vi "CRYUnflatten Data.vi"(11 "Unflatten data":string) -> (0 "Error?":bool, 2 "Datum":T2={"Name"="", "Curve"=[], "X data"=1, "Y data"=1, "Z data"=1, "X axis"=0, "Y axis"=1, "Z axis"=1, "X unit"="", "Y unit"="", "Z unit"="", "X dB ref"=1.0, "Y dB ref"=1.0, "Z dB ref"=1.0, "single val"=FALSE, "protected"=FALSE, "display X"=TRUE, "display Y"=FALSE, "display Z"=TRUE, "Test Info"="", "Step No."=0, "Plot Settings"={"Color"=0, "Interpolation"=0, "Point Style"=0, "Line Style"=0, "Point Color"=0, "Line Width"=0, "Bar Plot Style"=0, "Fill To"=0}, "AutoProtect"=FALSE} {"Z data" items=["dB", "Lin"]; "X data" items=["dB", "Lin"]; "Y data" items=["dB", "Lin"]; "Z dB ref" format="%.1f"; "Z axis" items=["Log", "Lin"]; "X dB ref" format="%.1f"; "X axis" items=["Log", "Lin"]; "Y axis" items=["Log", "Lin"]; "Y dB ref" format="%.1f"; "Curve"."z" format="%.2f"; "Curve"."y" format="%.2f"; "Curve"."x" format="%.2f"}, 3 "Header info":T1={"Data type"="Data            ", "Version"=1, "Dimensions"=0})   [LabVIEW 2013]
uses:
  Typedef Control/CRYData Cluster.ctl
  CRYCurveLibrary/Global/CRYCurve Library Global.vi
panel:
  # "-"
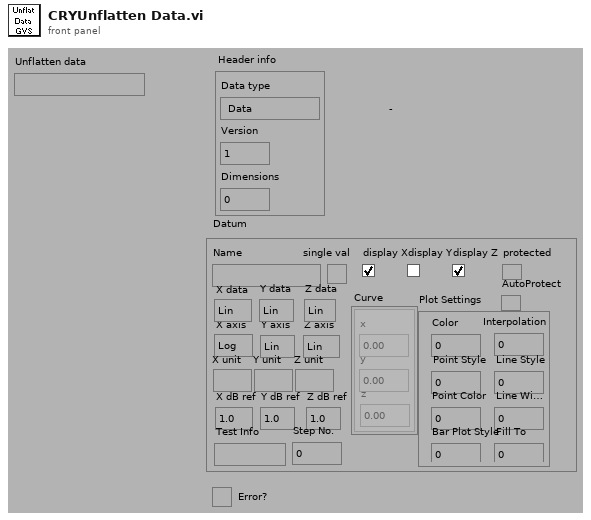
[diagram p1: front panel]
types:
  T1 = cluster{"Data type":string, "Version":u16, "Dimensions":u8}
  T2 = typedef "CRYData Cluster.ctl" = cluster{"Name":string, "Curve":cluster{"x":dbl, "y":dbl, "z":dbl}[], "X data":u16, "Y data":u16, "Z data":u16, "X axis":u16, "Y axis":u16, "Z axis":u16, "X unit":string, "Y unit":string, "Z unit":string, "X dB ref":dbl, "Y dB ref":dbl, "Z dB ref":dbl, "single val":bool, "protected":bool, "display X":bool, "display Y":bool, "display Z":bool, "Test Info":string, "Step No.":i32, "Plot Settings":cluster{"Color":u32, "Interpolation":u8, "Point Style":u8, "Line Style":u8, "Point Color":u32, "Line Width":u8, "Bar Plot Style":u8, "Fill To":i16}, "AutoProtect":bool}
  T3 = cluster{"Name":string, "Curve":cluster{"x":dbl, "y":dbl, "z":dbl}[], "X data":u16, "Y data":u16, "Z data":u16, "X axis":u16, "Y axis":u16, "Z axis":u16, "X unit":string, "Y unit":string, "Z unit":string, "X dB ref":dbl, "Y dB ref":dbl, "Z dB ref":dbl, "single val":bool, "protected":bool, "display X":bool, "display Y":bool, "display Z":bool, "Test Info":string, "Step No.":i32, "Plot Settings":cluster{"Color":u32, "Interpolation":u8, "Point Style":u8, "Line Style":u8, "Point Color":u32, "Line Width":u8, "Bar Plot Style":u8, "Fill To":i16}, "AutoProtect":bool}
  T4 = cluster{"unsigned byte array[0]":u8, "unsigned byte array[1]":u8, "unsigned byte array[2]":u8}
  T5 = cluster{"Name":string, "Curve":cluster{"x":dbl, "y":dbl, "z":dbl}[], "X data":u16, "Y data":u16, "Z data":u16, "X axis":u16, "Y axis":u16, "Z axis":u16, "X prefix":string, "Y prefix":string, "Z prefix":string, "X unit":string, "Y unit":string, "Z unit":string, "X dB ref":dbl, "Y dB ref":dbl, "Z dB ref":dbl}
  T6 = typedef "CRYData Cluster SC.ctl" = cluster{"Name":string, "Curve":cluster{"x":dbl, "y":dbl, "z":dbl}[], "X data":T7, "Y data":T7, "Z data":T7, "X axis":u16, "Y axis":u16, "Z axis":u16, "X unit":string, "Y unit":string, "Z unit":string, "X dB ref":dbl, "Y dB ref":dbl, "Z dB ref":dbl, "single val":bool, "protected":bool, "display X":bool, "display Y":bool, "display Z":bool, "Plot Settings":cluster{"Color":u32, "Interpolation":u8, "Point Style":u8, "Line Style":u8, "Point Color":u32, "Line Width":u8, "Bar Plot Style":u8, "Fill To":i16}, "Test Info":string}
  T7 = typedef "CRYAxis Unit Type.ctl" = u16
  T8 = cluster{"Color":u32, "Interpolation":u8, "Point Style":u8, "Line Style":u8, "Point Color":u32, "Line Width":u8, "Bar Plot Style":u8, "Fill To":i16}
  T9 = cluster{"substring":string, u16, "unsigned byte array[2]":u8}
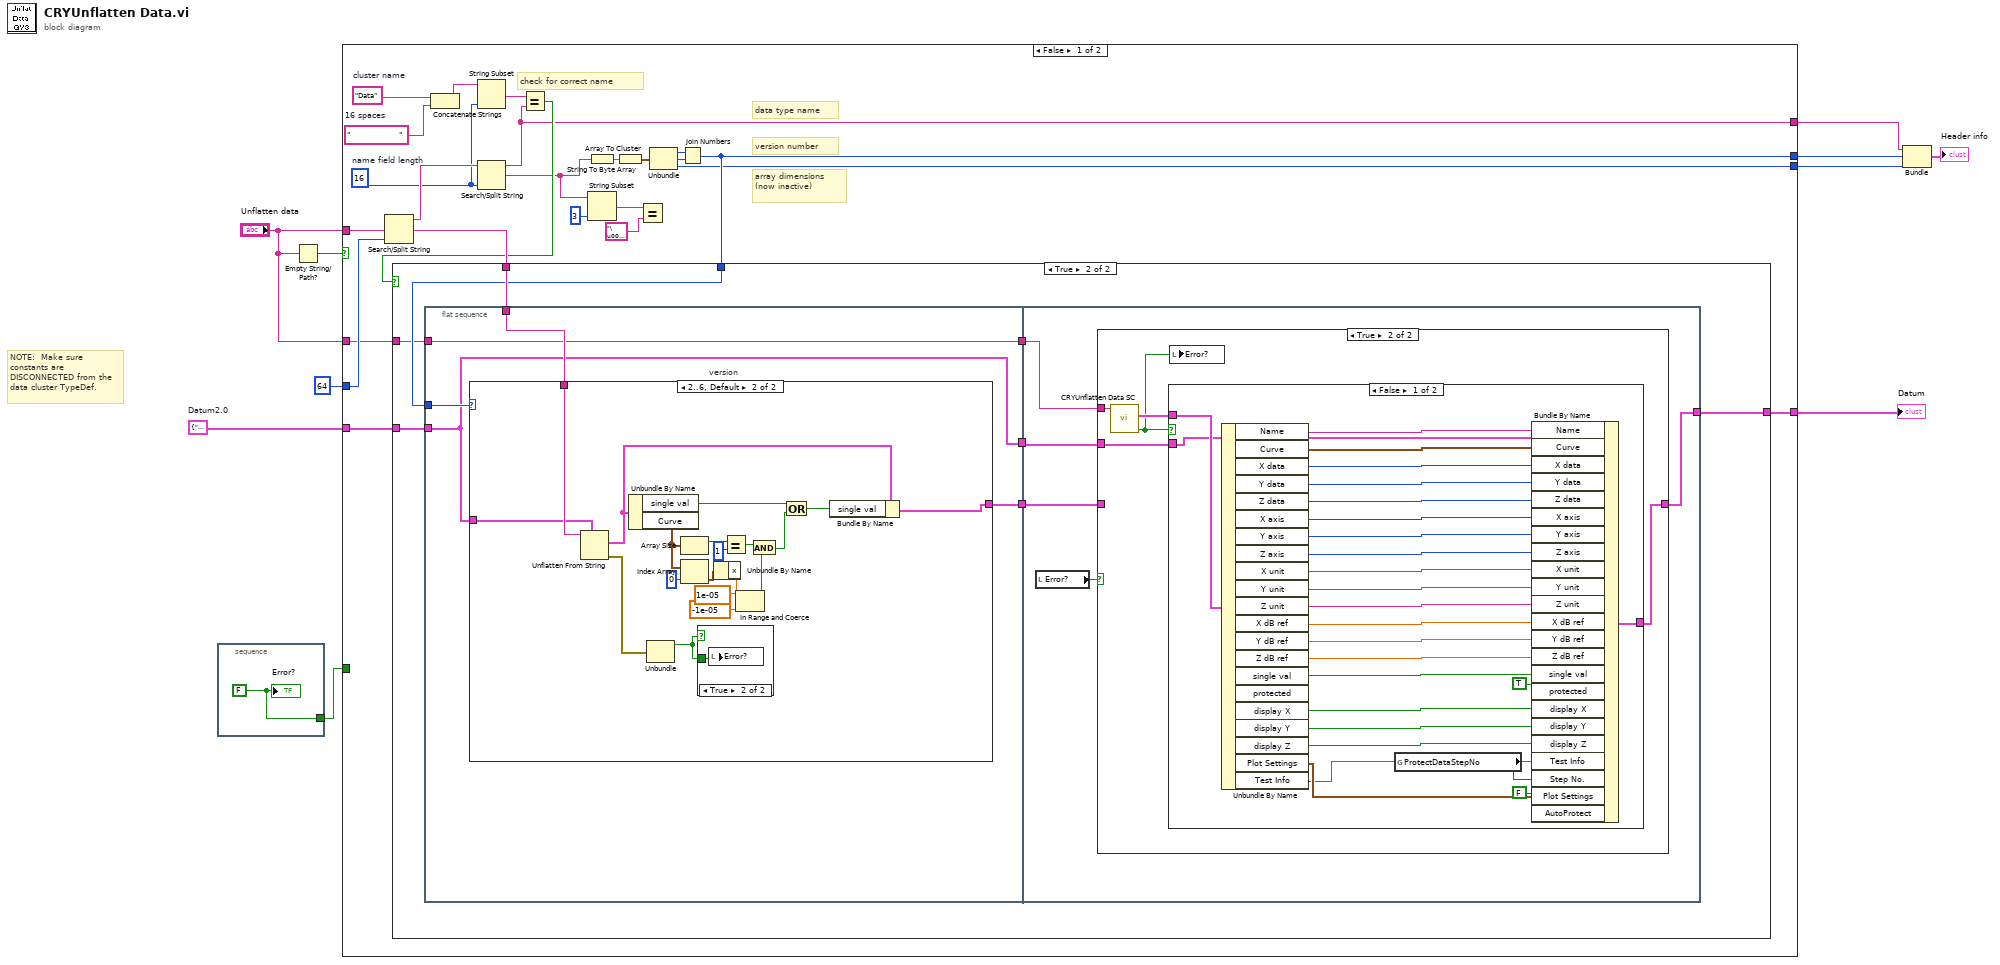
[diagram p0: block diagram]
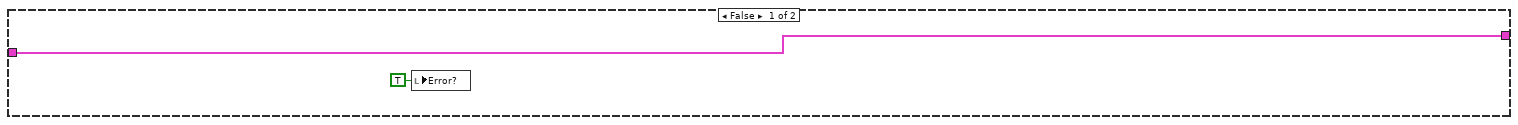
[diagram p2: hidden frame]
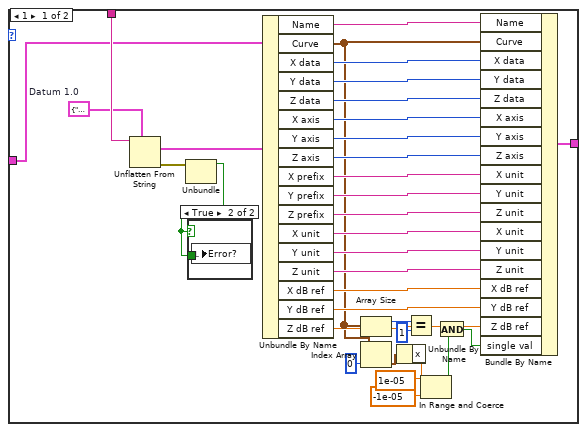
[diagram p3: hidden frame]
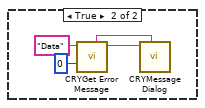
[diagram p7: hidden frame]
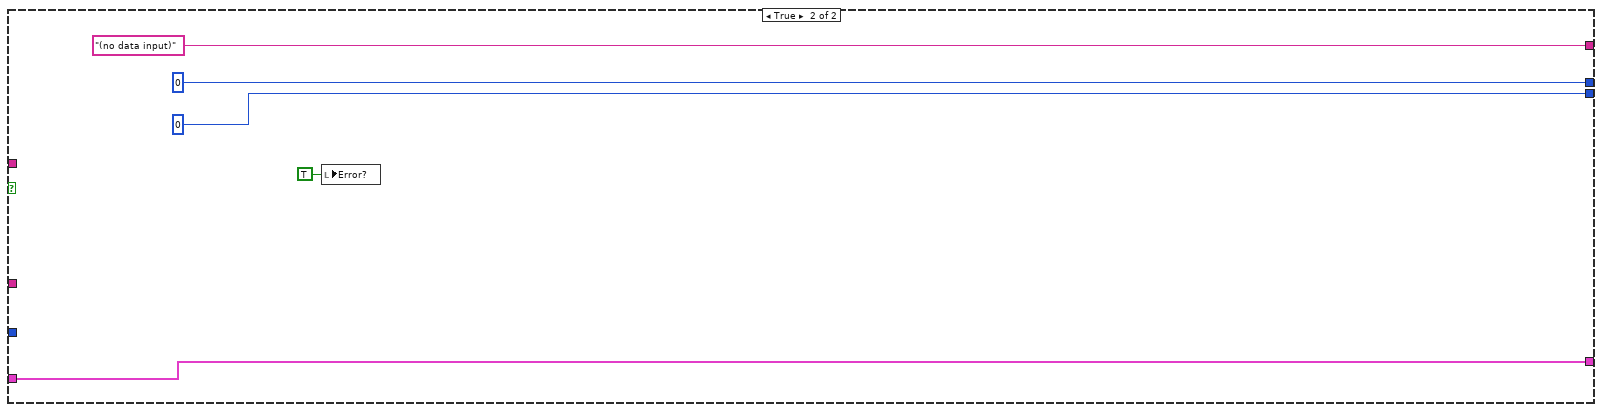
[diagram p8: hidden frame]
diagram:
  w2 = T3 {"Name"="", "Curve"=[], "X data"=1, "Y data"=1, "Z data"=1, "X axis"=0, "Y axis"=1, "Z axis"=1, "X unit"="", "Y unit"="", "Z unit"="", "X dB ref"=1.0, "Y dB ref"=1.0, "Z dB ref"=1.0, "single val"=FALSE, "protected"=FALSE, "display X"=TRUE, "display Y"=TRUE, "display Z"=TRUE, "Test Info"="", "Step No."=0, "Plot Settings"={"Color"=0, "Interpolation"=0, "Point Style"=0, "Line Style"=0, "Point Color"=0, "Line Width"=0, "Bar Plot Style"=0, "Fill To"=0}, "AutoProtect"=FALSE}  # Datum2.0
  # "NOTE:  Make sure constants are DISCONNECTED from the data cluster TypeDef."
  n1 = stacked-sequence {
    tunnel: [w11] -> w4
    frame #0 {
      w11 = FALSE
      "Error?" <- w11
    }
  }
  n2 = Empty String/Path?(string/path="Unflatten data") -> (empty?=w10:bool)
  n3 = case shown="False" w10 {
    tunnel: "Unflatten data" -> [w35 _]
    tunnel: 64 ("header length") -> [w29 _]
    tunnel: [w26 u16 0] -> w7
    tunnel: [w19 u8 0] -> w8
    tunnel: [w20 "(no data input)" ("substring")] -> w6
    tunnel: w4 -> [_ _]
    tunnel: [w18 w147] -> w3
    tunnel: w2 -> [w17 w147]
    tunnel: "Unflatten data" -> [w16 _]
    frame False {
      w24 = "                "  # 16 spaces
      w25 = "Data"  # cluster name
      w22 = 16  # name field length
      # "check for correct name"
      # "array dimensions\n(now inactive)"
      # "version number"
      # "data type name"
      n4 = Search/Split String(string=w35, offset (0)=w29) -> (substring before match=w28:string, match + rest of string=w30:string)  [unwired: 2 out]
      n5 = Concatenate Strings(w25, w24) -> (w23:string)
      n6 = String Subset(string=w23, length (rest)=w22) -> (substring=w21:string)  [unwired: 1 out]
      n7 = Search/Split String(string=w28, offset (0)=w22) -> (substring before match=w20:string, match + rest of string=w15:string)  [unwired: 2 out]
      n8 = Equal?(x=w21, y=w20) -> (x = y?=w27:bool)
      n9 = String To Byte Array(string=w15) -> (unsigned byte array=w34:u8[])
      n10 = String Subset(string=w15, length (rest)=3 ("name field length")) -> (substring=w13:string)  [unwired: 1 out]
      n11 = Array To Cluster(array=w34) -> (cluster=w33:T4)
      n12 = Equal?(x=w13, y="\u0000\u0006\u0000" ("concatenated string")) -> ()  [unwired: 1 out]
      n13 = Unbundle(w33) -> ("unsigned byte array[0]"=w32:u8, "unsigned byte array[1]"=w31:u8, "unsigned byte array[2]"=w19:u8)
      n14 = Join Numbers(hi=w32, lo=w31) -> ((hi.lo)=w26:u16)
      n15 = case shown="True" w27 {
        tunnel: w30 -> [_ w45]
        tunnel: w26 -> [_ w44]
        tunnel: [w36 w42] -> w18
        tunnel: w17 -> [w36 w43]
        tunnel: w16 -> [_ w41]
        frame False {
          n16 = local write "Error?"(TRUE ("Error?")) -> ()
        }
        frame True {
          n17 = flat-sequence {
            tunnel: w45 -> [w50]
            tunnel: w44 -> [w49]
            tunnel: w43 -> [w48]
            tunnel: [w48] -> w40
            tunnel: w41 -> [w46]
            tunnel: [w46] -> w39
            tunnel: [w47] -> w38
            tunnel: w40 -> [w110]
            tunnel: [w106] -> w42
            tunnel: w39 -> [w109]
            tunnel: w38 -> [w107]
            frame #0 {
              n18 = case "version" shown="2..6, Default" w49 {
                tunnel: w50 -> [w84 w104]
                tunnel: [w83 w89] -> w47
                tunnel: w48 -> [w52 w102]
                frame 1 {
                  w81 = T5 {"Name"="", "Curve"=[], "X data"=0, "Y data"=0, "Z data"=0, "X axis"=0, "Y axis"=0, "Z axis"=0, "X prefix"="", "Y prefix"="", "Z prefix"="", "X unit"="", "Y unit"="", "Z unit"="", "X dB ref"=0.0, "Y dB ref"=0.0, "Z dB ref"=0.0}  # Datum 1.0
                  n19 = Unflatten From String(type=w81, binary string=w84) -> (value=w80:T5, error out=w51:errorcluster)  [unwired: 1 in, 3 out]
                  n20 = Unbundle(w51) -> ("status"=w82:bool)  [unwired: 2 out]
                  n21 = case shown="True" w82 {
                    tunnel: w82 -> [_ w85]
                    frame False {
                    }
                    frame True {
                      n22 = local write "Error?"(w85) -> ()
                    }
                  }
                  n23 = Unbundle By Name(w80) -> ("Name"=w79:string, "Curve"=w53:cluster{"x":dbl, "y":dbl, "z":dbl}[], "X data"=w78:u16, "Y data"=w77:u16, "Z data"=w76:u16, "X axis"=w75:u16, "Y axis"=w74:u16, "Z axis"=w73:u16, "X prefix"=w72:string, "Y prefix"=w71:string, "Z prefix"=w70:string, "X unit"=w69:string, "Y unit"=w68:string, "Z unit"=w67:string, "X dB ref"=w66:dbl, "Y dB ref"=w65:dbl, "Z dB ref"=w64:dbl)
                  n24 = Array Size(array=w53) -> (size(s)=w60:i32)
                  n25 = Index Array(array=w53, index=0 ("Index")) -> (element=w57:cluster{"x":dbl, "y":dbl, "z":dbl})
                  n26 = Unbundle By Name(w57) -> ("x"=w56:dbl)
                  n27 = Equal?(x=w60, y=1) -> (x = y?=w58:bool)
                  n28 = In Range and Coerce(upper limit=1e-05, x=w56, lower limit=-1e-05) -> (In Range?=w55:bool)  [unwired: 1 out]
                  n29 = And(x=w58, y=w55) -> (x .and. y?=w54:bool)
                  n30 = Bundle By Name(cluster=w52, "Name"=w79, "Curve"=w53, "X data"=w78, "Y data"=w77, "Z data"=w76, "X axis"=w75, "Y axis"=w74, "Z axis"=w73, "X unit"=w72, "Y unit"=w71, "Z unit"=w70, "X unit"=w69, "Y unit"=w68, "Z unit"=w67, "X dB ref"=w66, "Y dB ref"=w65, "Z dB ref"=w64, "single val"=w54) -> (w83:T3)
                }
                frame 2..6, Default {
                  n31 = Unflatten From String(type=w102, binary string=w104) -> (value=w90:T3, error out=w101:errorcluster)  [unwired: 1 in, 3 out]
                  n32 = Unbundle By Name(w90) -> ("single val"=w88:bool, "Curve"=w91:cluster{"x":dbl, "y":dbl, "z":dbl}[])
                  n33 = Unbundle(w101) -> ("status"=w103:bool)  [unwired: 2 out]
                  n34 = Array Size(array=w91) -> (size(s)=w97:i32)
                  n35 = Index Array(array=w91, index=0 ("Index")) -> (element=w94:cluster{"x":dbl, "y":dbl, "z":dbl})
                  n36 = case shown="True" w103 {
                    tunnel: w103 -> [_ w105]
                    frame False {
                    }
                    frame True {
                      n37 = local write "Error?"(w105) -> ()
                    }
                  }
                  n38 = Unbundle By Name(w94) -> ("x"=w93:dbl)
                  n39 = Equal?(x=w97, y=1) -> (x = y?=w95:bool)
                  n40 = In Range and Coerce(upper limit=1e-05, x=w93, lower limit=-1e-05) -> (In Range?=w92:bool)  [unwired: 1 out]
                  n41 = And(x=w95, y=w92) -> (x .and. y?=w87:bool)
                  n42 = Or(x=w88, y=w87) -> (x .or. y?=w86:bool)
                  n43 = Bundle By Name(cluster=w90, "single val"=w86) -> (w89:T3)
                }
              }
            }
            frame #1 {
              n44 = local read "Error?"() -> (w108:bool)
              n45 = case shown="True" w108 {
                tunnel: w110 -> [_ w114]
                tunnel: w109 -> [_ w113]
                tunnel: w107 -> [w111 _]
                tunnel: [w111 w112] -> w106
                frame False {
                }
                frame True {
                  n46 = call "CRYUnflatten Data SC.vi"("Unflatten data"=w113) -> ("Error?"=w115:bool, "Data out"=w116:T6)  [unwired: 7 in, 1 out]
                  n47 = case shown="False" w115 {
                    tunnel: w116 -> [w142 _]
                    tunnel: w114 -> [w141 _]
                    tunnel: [w132 _] -> w112
                    frame False {
                      n48 = Unbundle By Name(w142) -> ("Name"=w140:string, "Curve"=w139:cluster{"x":dbl, "y":dbl, "z":dbl}[], "X data"=w138:T7, "Y data"=w137:T7, "Z data"=w136:T7, "X axis"=w135:u16, "Y axis"=w134:u16, "Z axis"=w133:u16, "X unit"=w131:string, "Y unit"=w130:string, "Z unit"=w129:string, "X dB ref"=w128:dbl, "Y dB ref"=w127:dbl, "Z dB ref"=w126:dbl, "single val"=w125:bool, "display X"=w124:bool, "display Y"=w123:bool, "display Z"=w122:bool, "Plot Settings"=w121:T8, "Test Info"=w120:string)  [unwired: 1 out]
                      n49 = global read "CRYCurve Library Global.vi" "ProtectDataStepNo"() -> (w117:i32)
                      n50 = Bundle By Name(cluster=w141, "Name"=w140, "Curve"=w139, "X data"=w138, "Y data"=w137, "Z data"=w136, "X axis"=w135, "Y axis"=w134, "Z axis"=w133, "X unit"=w131, "Y unit"=w130, "Z unit"=w129, "X dB ref"=w128, "Y dB ref"=w127, "Z dB ref"=w126, "single val"=w125, "protected"=TRUE, "display X"=w124, "display Y"=w123, "display Z"=w122, "Test Info"=w120, "Step No."=w117, "Plot Settings"=w121, "AutoProtect"=FALSE) -> (w132:T3)
                    }
                    frame True {
                      n51 = call "CRYGet Error Message.vi"("Error No"=0, "Kind"="Data") -> ("Message"=w144:string, "Window Title"=w143:string)  [unwired: 4 in, 4 out]
                      n52 = call "CRYMessage Dialog.vi"("Window Title"=w143, "Message Content"=w144) -> ()  [unwired: 8 in, 2 out]
                    }
                  }
                  n53 = local write "Error?"(w115) -> ()
                }
              }
            }
          }
        }
      }
    }
    frame True {
      n54 = local write "Error?"(TRUE ("Error?")) -> ()
    }
  }
  "Datum" <- w3
  n55 = Bundle("substring"=w6, w7, "unsigned byte array[2]"=w8) -> (→"Header info":T9)  [unwired: 1 out]
